vi "CalcAngle.vi"(8 "XY b":cluster{dbl, dbl}, 9 "XY a":cluster{dbl, dbl}, 11 "Draw Area Size":T1) -> (1 "Angle (deg)":sgl, 3 "Angle (rad)":sgl)   [LabVIEW 2021]
uses:
  <vilib>/Utility/miscctls.llb/LVBoundsTypeDef.ctl
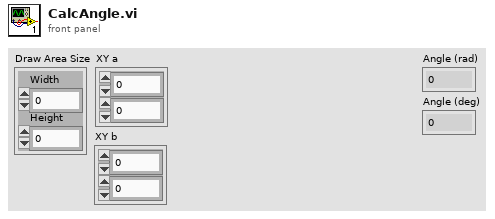
[diagram p1: front panel]
types:
  T1 = typedef "LVBoundsTypeDef.ctl" = cluster{"Width":u32, "Height":u32}
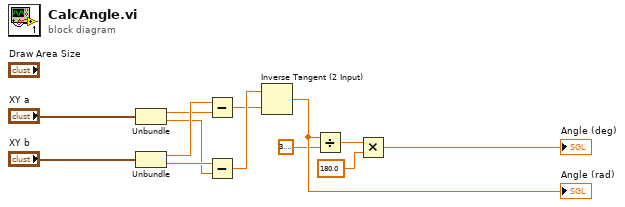
[diagram p0: block diagram]
diagram:
  n1 = Unbundle("XY a") -> (w8:dbl, w4:dbl)
  n2 = Unbundle("XY b") -> (w9:dbl, w5:dbl)
  n3 = Subtract(x=w9, y=w8) -> (x-y=w6:dbl)
  n4 = Subtract(x=w5, y=w4) -> (x-y=w7:dbl)
  n5 = Inverse Tangent (2 Input)(1:w6, 2:w7) -> (0:w13:dbl)
  "Angle (rad)" <- w13
  n6 = Divide(x=w13, y=3.141592653589793) -> (x/y=w2:dbl)
  n7 = Multiply(x=w2, y=180.0) -> (x*y=→"Angle (deg)":dbl)
